vi "Dequeue Job.vi"(8 "error in (no error)":errorcluster, 9 "timeout in ms (-1)":i32=-1, 11 "Mock Worker in":refnum<class "Mock Work Dispatcher.lvclass">) -> (0 "error out":errorcluster, 1 "timed out?":bool, 2 "element":refnum<class>, 3 "Mock Worker out":refnum<class "Mock Work Dispatcher.lvclass">)   [LabVIEW 2020, in "Mock Work Dispatcher.lvclass"]
uses:
  Mock Work Dispatcher.lvclass
  Mock Work Dispatcher.lvclass/Mock Work Dispatcher.ctl
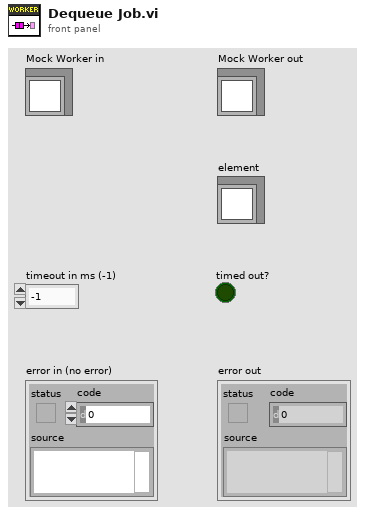
[diagram p1: front panel]
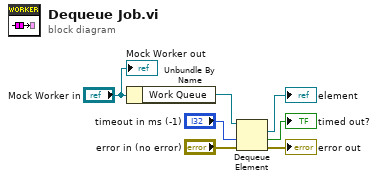
[diagram p0: block diagram]
diagram:
  n1 = Unbundle By Name("Mock Worker in") -> ("Work Queue"=w4:refnum<queue>)
  n2 = Dequeue Element(queue=w4, timeout in ms (-1)="timeout in ms (-1)", error in (no error)="error in (no error)") -> (element=→"element":refnum<class>, timed out?=→"timed out?":bool, error out=→"error out":errorcluster)  [unwired: 1 out]
  "Mock Worker out" <- "Mock Worker in"
